vi "Accelerometer Logger.vi"() -> ()   [LabVIEW 2012]
uses:
  Accelerometer Data.ctl
  <vilib>/Platform/TimedLoop/XDataNode/timing_clust.ctl
  <vilib>/Platform/TimedLoop/XDataNode/nitl_modes.ctl
  <vilib>/Platform/TimedLoop/XDataNode/wakeup.ctl
  <vilib>/Analysis/_algsub.llb/Real Vector Norm.vi
  <vilib>/platform/TimedLoop/XDataNode/XDataNode.xnode
  <vilib>/Platform/TimedLoop/XDataNode/XDNodeRunTimeDep.lvlib
  <vilib>/Analysis/NI_AALPro.lvlib
panel:
  out "Trigger":bool
  out "mag":dbl(slide) caption="Magnitude (g)" scale=0.0..2.0
  in  "Stop":bool
  in  "accel range (g)":u16(ring)=2 items=["2"=2, "4"=4, "8"=8, "16"=16]
  in  "gyro range (deg/sec)":u16(ring)=250 items=["250"=250, "500"=500, "1000"=1000, "2000"=2000]
  out "Gyro":waveform(dbl)[](graph)
  out "Accel":waveform(dbl)[](graph)
  in  "Sampling rate":dbl[unit]=100.0
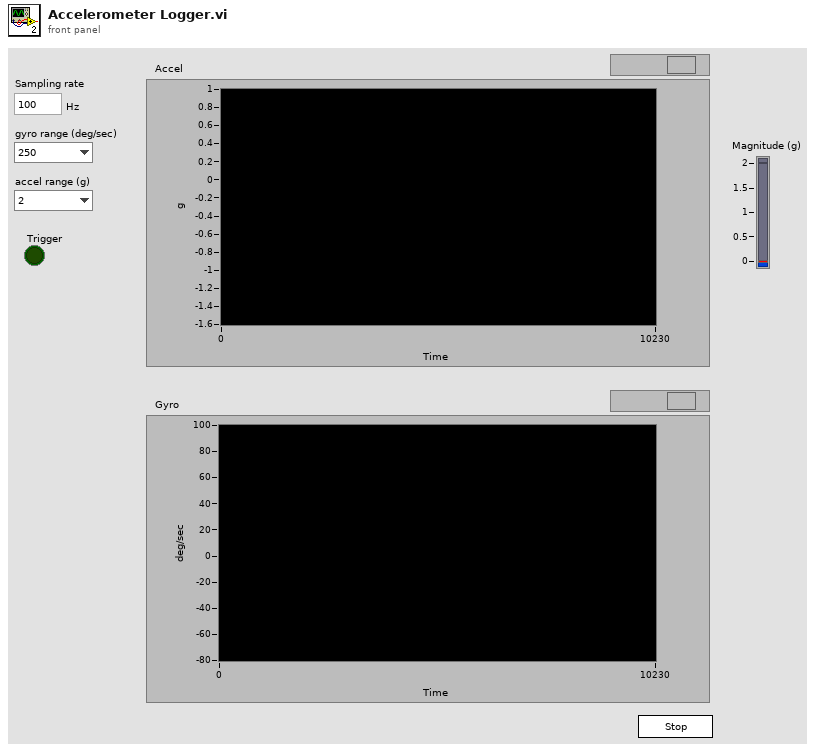
[diagram p1: front panel]
types:
  T1 = typedef "Accelerometer Data.ctl" = cluster{"Accel":dbl[], "Gyro":dbl[], "Time":u64, "Trigger":bool}
  T2 = typedef "Accelerometer.ctl" = cluster{"Device":T3, "i2c configuration":T4}
  T3 = typedef "ni845xControl.ctl" = refnum<k21>
  T4 = typedef "ni845xI2cConfiguration.ctl" = refnum<k20>
  T5 = typedef "XDNodeRunTimeDep.lvlib/timing_clust.ctl" = cluster{"Expected End [f-1]":u64, "Actual End [f-1]":u64, "Finished Late? [f-1]":bool, "Expected End [i-1]":u64, "Actual End [i-1]":u64, "Finished Late? [i-1]":bool, "Expected Start [i]":u64, "Actual Start [i]":u64, "Expected Start [f]":u64, "Actual Start [f]":u64, "Source Name":string, "Structure Name":string, "Period":i64, "Deadline":i64, "Offset":i64, "Start":i64, "Priority":i32, "Timeout":i32, "Mode":T6, "Wakeup Reason":T7, "Error":errorcluster, "Source Type":string, "Secondary Source Type":string, "Global End Time":u64, "Global Start Time":u64, "Frame Duration":u64, "Iteration Duration":u64, "Assigned CPU":i32, "I/O Scan Engine Mode":u32}
  T6 = typedef "XDNodeRunTimeDep.lvlib/nitl_modes.ctl" = enum32{"No Change", "Process missed periods, maintain original phase", "Discard missed periods, maintain original phase", "Process missed periods, ignore original phase", "Discard missed periods, ignore original phase"}
  T7 = typedef "XDNodeRunTimeDep.lvlib/wakeup.ctl" = enum32{"Normal", "Aborted", "Asynchronous wakeup", "Timing source error", "Timed loop error", "Timeout"}
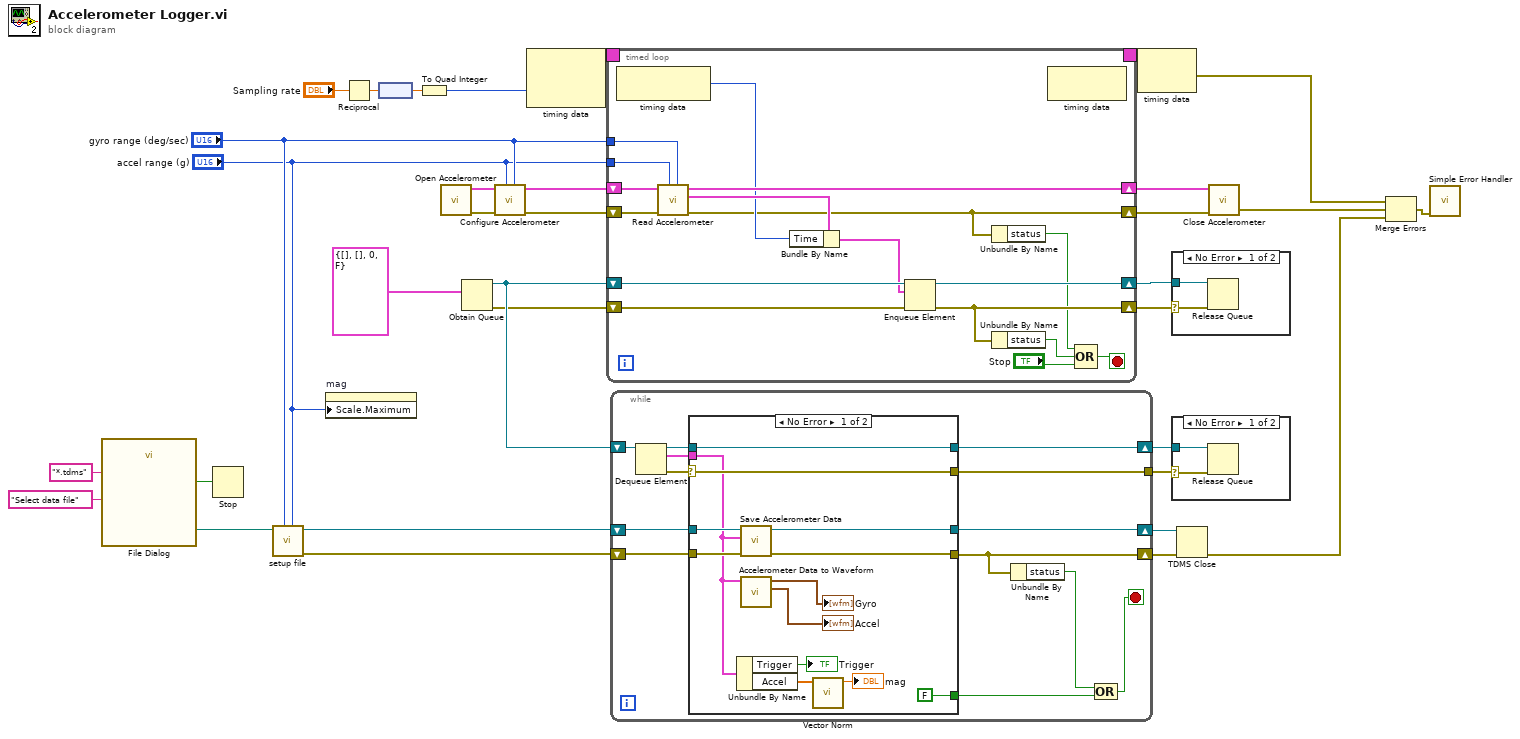
[diagram p0: block diagram]
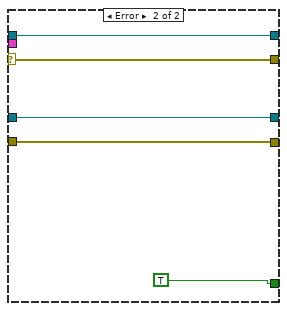
[diagram p4: hidden frame]
diagram:
  n1 = call "File Dialog"("prompt"="Select data file", "pattern (all files)"="*.tdms") -> ("selected path"=w16:path, "cancelled"=w15:bool)  [unwired: 10 in, 2 out]
  n2 = Stop(stop? (T)=w15) -> ()
  n3 = call "setup file.vi"("accel range"="accel range (g)", "gyro range"="gyro range (deg/sec)", "selected path"=w16) -> ("error out"=w12:errorcluster, "tdms file out"=w13:refnum<k34>)  [unwired: 6 in, 1 out]
  n4 = property on="mag" class="Slide (strict)"("Scale.Maximum"="accel range (g)") -> ()  [unwired: 2 in, 2 out]
  n5 = Reciprocal(x="Sampling rate") -> (1/x=w30:dbl[unit])
  n6 = node(w30) -> (w29:dbl)
  n7 = To Quad Integer(1:w29) -> (0:w28:i64)
  n8 = call "Open Accelerometer.vi"() -> ("error out"=w27:errorcluster, "Accelerometer"=w26:T2)  [unwired: 10 in]
  n9 = Obtain Queue(element data type=T1 {"Accel"=[], "Gyro"=[], "Time"=0, "Trigger"=FALSE} ("Accelerometer Data")) -> (queue out=w24:refnum<queue>, error out=w23:errorcluster)  [unwired: 4 in, 1 out]
  n10 = call "Configure Accelerometer.vi"("gyro range (deg/sec)"="gyro range (deg/sec)", "accel range (g)"="accel range (g)", "error in (no error)"=w27, "Accelerometer"=w26) -> ("error out"=w21:errorcluster, "Accelerometer out"=w22:T2)  [unwired: 6 in]
  n11 = node-c288(w28) -> (w33:T5)  [unwired: 1 in]
  n12 = timed-loop {
    timing: w33 -> [_]
    timing-out: [_] -> w32
    tunnel: "accel range (g)" -> [w48]
    tunnel: "gyro range (deg/sec)" -> [w47]
    shift-right: [w37] -> w6
    shift-left: w23 -> [w44]
    shift-right: [w35] -> w19
    shift-left: w21 -> [w49]
    shift-right: [w43] -> w7
    shift-left: w24 -> [w45]
    shift-right: [w46] -> w20
    shift-left: w22 -> [w50]
    stop <- w39 stop-if-true
    n13 = node-c288() -> (w40:i64)  [unwired: 1 in]
    n14 = call "Read Accelerometer.vi"("gyro range (deg/sec)"=w47, "accel range (g)"=w48, "error in (no error)"=w49, "Accelerometer"=w50) -> ("error out"=w35:errorcluster, "Accelerometer Data"=w42:T1, "Accelerometer out"=w46:T2)  [unwired: 4 in, 1 out]
    n15 = Bundle By Name(cluster=w42, "Time"=w40) -> (w41:T1)
    n16 = Enqueue Element(queue=w45, element=w41, error in (no error)=w44) -> (queue out=w43:refnum<queue>, error out=w37:errorcluster)  [unwired: 1 in, 1 out]
    n17 = Unbundle By Name(w35) -> ("status"=w34:bool)
    n18 = Unbundle By Name(w37) -> ("status"=w36:bool)
    n19 = node-c288() -> ()  [unwired: 1 in, 1 out]
    n20 = Compound Arithmetic op=OR(w34, w36, "Stop") -> (w39:bool)
  }
  n21 = while {
    shift-right: [w61] -> w8
    shift-left: w24 -> [w66]
    shift-right: [w59] -> w10
    shift-left: w13 -> [w63]
    shift-right: [w56] -> w11
    shift-left: w12 -> [w62]
    tunnel: [w54] -> w9
    stop <- w58 stop-if-true
    n22 = Dequeue Element(queue=w66) -> (queue out=w60:refnum<queue>, element=w64:T1, error out=w65:errorcluster)  [unwired: 2 in, 1 out]
    n23 = case shown="No Error" w65 {
      selector: w65 -> [w71 w80]
      tunnel: w64 -> [w70 _]
      tunnel: [FALSE TRUE] -> w57
      tunnel: w63 -> [w77 w82]
      tunnel: w62 -> [w76 w81]
      tunnel: [w75 w82] -> w59
      tunnel: [w74 w81] -> w56
      tunnel: [w73 w83] -> w61
      tunnel: w60 -> [w73 w83]
      tunnel: [w71 w80] -> w54
      frame No Error {
        n24 = Unbundle By Name(w70) -> ("Trigger"=→"Trigger":bool, "Accel"=w69:dbl[])
        n25 = call "Save Accelerometer Data.vi"("error in (no error)"=w76, "Accelerometer Data"=w70, "tdms file"=w77) -> ("error out"=w74:errorcluster, "tdms file out"=w75:refnum<k34>)  [unwired: 7 in]
        n26 = call "Accelerometer Data to Waveform.vi"("Accelerometer Data"=w70) -> ("accel plot"=→"Accel":waveform(dbl)[], "gyro plot"=→"Gyro":waveform(dbl)[])  [unwired: 9 in]
        n27 = call-poly <vilib>:"Vector Norm.vi"("Input Vector"=w69) -> ("norm"=→"mag":dbl)  [unwired: 9 in, 1 out]
      }
      frame Error {
      }
    }
    n28 = Unbundle By Name(w56) -> ("status"=w55:bool)
    n29 = Compound Arithmetic op=OR(w55, w57) -> (w58:bool)
  }
  n30 = node-c288(w32) -> (w1:errorcluster)
  n31 = case shown="No Error" w6 {
    selector: w6 -> [w85 _]
    tunnel: w7 -> [w86 _]
    frame No Error {
      n32 = Release Queue(queue=w86, error in (no error)=w85) -> ()  [unwired: 1 in, 3 out]
    }
    frame Error {
    }
  }
  n33 = case shown="No Error" w9 {
    selector: w9 -> [w87 _]
    tunnel: w8 -> [w88 _]
    frame No Error {
      n34 = Release Queue(queue=w88, error in (no error)=w87) -> ()  [unwired: 1 in, 3 out]
    }
    frame Error {
    }
  }
  n35 = TDMS Close(8:w11, 11:w10) -> (0:w3:errorcluster)  [unwired: 1 out]
  n36 = call "Close Accelerometer.vi"("error in (no error)"=w19, "Accelerometer"=w20) -> ("error out"=w4:errorcluster)  [unwired: 9 in]
  n37 = Merge Errors(w1, w4, w3) -> (w5:errorcluster)
  n38 = call <vilib>:"Simple Error Handler.vi"("error in (no error)"=w5) -> ()  [unwired: 4 in, 5 out]
